vi "Projeto.vi"(8 "Error In":errorcluster) -> (0 "Error Out":errorcluster)   [LabVIEW 2014]
uses:
  Aquisicao de Dados.lvlib
  <vilib>/express/express analysis/Spectral/XNode/ExpressSpectralMeasurementsBlockNode.xnode
  <vilib>/express/express analysis/Spectral/Block/exnSpectralBlock spectral measurements RMS poly.vi
  <vilib>/express/express analysis/Spectral/Block/exnSpectralBlock spectral measurements RMS WFM.vi
  <vilib>/measure/NI_MAPro.lvlib
  <vilib>/measure/matone.llb/Extract Multiple Tone Information 1 Chan.vi
panel:
  out "resolução espectral":dbl
  out "V/2^n":dbl
  out "Período de amostragem":dbl
  out "multiple tone information":T1(array[cluster]) {"detected phase (deg)" format="%_6g"; "detected amplitude" format="%_6p"; "detected frequency" format="%_6p"}
  out "frequência de amostragem":dbl
  out "período de amostragem":dbl
  out "amostras janelada":i32
  out "amostras total":i32
  out "Waveform Graph 3":cluster{"f0":dbl, "df":dbl, "magnitude":dbl[]}(graph)
  out "mín local":dbl
  out "máx local":dbl
  out "min global":dbl
  out "max global":dbl
  out "Waveform Graph 2":cluster{"f0":dbl, "df":dbl, "magnitude":dbl[]}(graph)
  out "Waveform Graph":waveform(dbl)(graph)
  in  "stop":bool
  out "Canal 1":waveform(dbl)(graph)
  out "Canal 0":waveform(dbl)(graph)
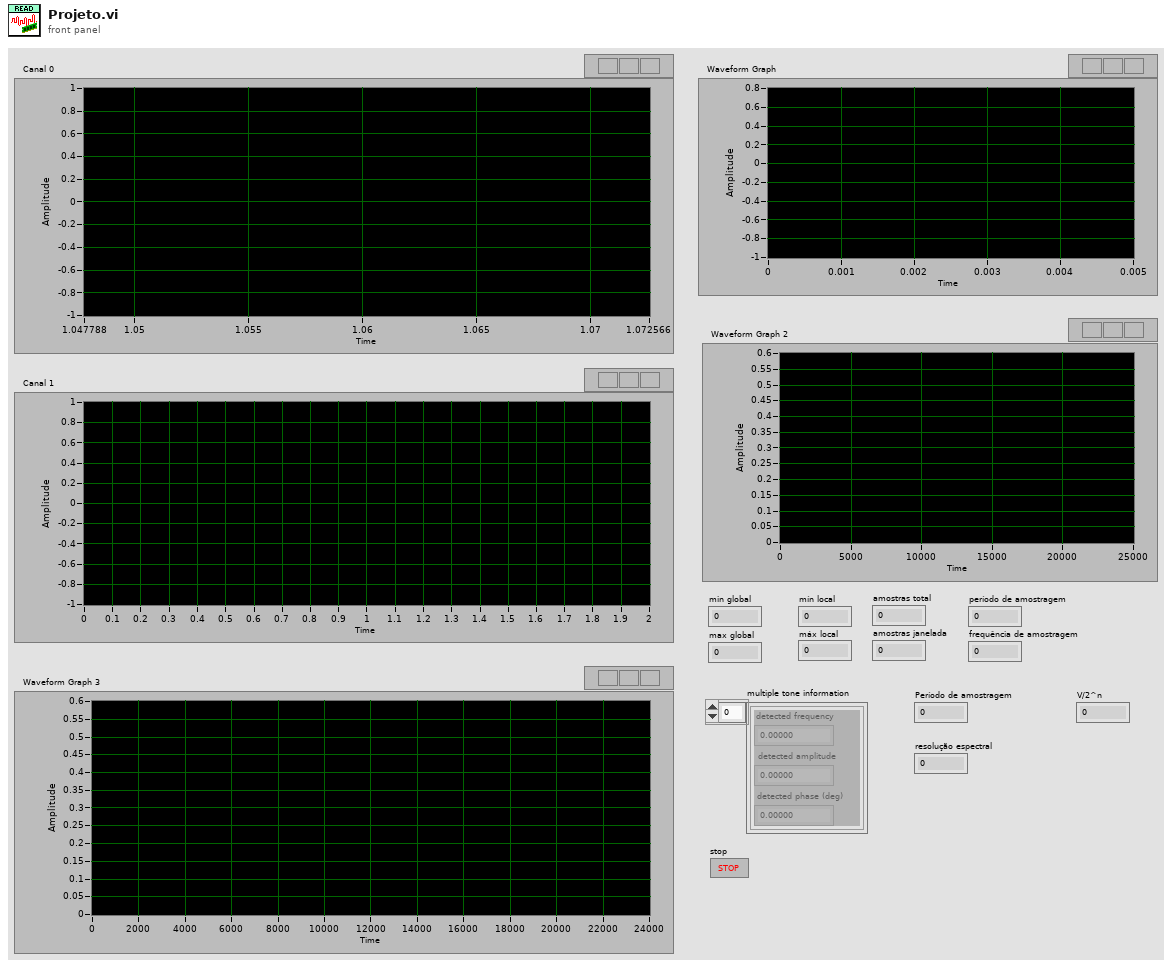
[diagram p1: front panel]
types:
  T1 = cluster{"detected frequency":dbl, "detected amplitude":dbl, "detected phase (deg)":dbl}[]
  T2 = enum32{".WAV File", "LTSpice Simulation", "Microphone", "MultiSim Simulation", "Serial Port"}
  T3 = typedef "Aquisicao de Dados.lvlib/_ACC_DATA_ Config DAta State.ctl" = cluster{"_RAW_ Traces":cluster{"Trace Name":string, "Trace Type":string, "Trace Raw Data":dbl[], "Trace Waveform":waveform(dbl)}[], "_WAV_ Traces":waveform(dbl)[], "_MIC_ Config":cluster{"task ID":T4, "Data Chunk Size":i32, "Num Channels":i32, "Resolution":i32, "Sampling Frequency":dbl, "device ID":u32, "Num Chunks":i32}, "_LVM_ Traces":cluster{"Trace Name":string, "Trace Type":string, "Trace Raw Data":dbl[], "Trace Waveform":waveform(dbl)}[]}
  T4 = typedef "Sound Input Task ID.ctl" = u32
  T5 = cluster{"averaging mode":u16, "weighting mode":u16, "number of averages":u32}
  T6 = cluster{"dB On (F)":bool, "unwrap phase (F)":bool, "convert to degree (F)":bool}
  T7 = typedef "LVCursorListTypeDef.ctl" = cluster{"Name":string, "Color":u32, "Style":u8, "Point Style":u8, "Name Visible":bool, "Allow Drag":bool, "Cursor Mode":u32, "Plot":i32, "Index":i32, "Position":cluster{"X":dbl, "Y":dbl}, "X Scale":u32, "Y Scale":u32, "Watch Plots":i32[], "Watch All Plots":bool, "Plot Area":i32, "Label Offset":cluster{"X":dbl, "Y":dbl}}[]
  T8 = cluster{"Name":string, "Color":u32, "Style":u8, "Point Style":u8, "Name Visible":bool, "Allow Drag":bool, "Cursor Mode":u32, "Plot":i32, "Index":i32, "Position":cluster{"X":dbl, "Y":dbl}, "X Scale":u32, "Y Scale":u32, "Watch Plots":i32[], "Watch All Plots":bool, "Plot Area":i32, "Label Offset":cluster{"X":dbl, "Y":dbl}}
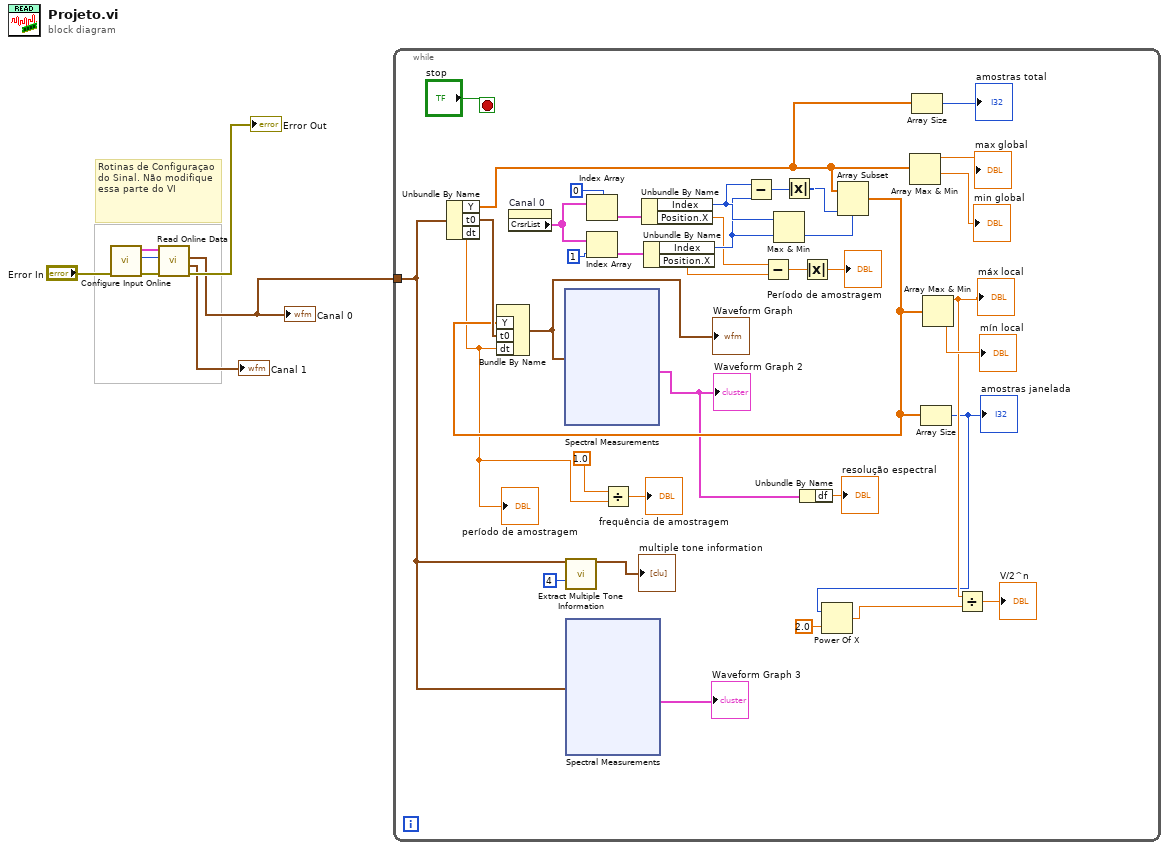
[diagram p0: block diagram]
diagram:
  # "Rotinas de Configuraçao do Sinal. Não modifique essa parte do VI"
  n1 = call "Configure Input Online.vi"("Error In"="Error In") -> ("Error Out"=w7:errorcluster, "Metodo de Entrada"=w5:T2, "Config Out"=w3:T3)  [unwired: 8 in]
  n2 = call "Read Online Data.vi"("Error In"=w7, "Metodo de Entrada"=w5, "Config Out"=w3) -> ("Error Out"=→"Error Out":errorcluster, "Channel 1"=→"Canal 1":waveform(dbl), "Channel 0"=w1:waveform(dbl))  [unwired: 6 in]
  "Canal 0" <- w1
  n3 = while {
    tunnel: w1 -> [w24]
    stop <- "stop" stop-if-true
    n4 = Unbundle By Name(w24) -> ("Y"=w29:dbl[], "t0"=w43:timestamp, "dt"=w26:dbl)
    "período de amostragem" <- w26
    n5 = property on="Canal 0" class="WFGraph (strict)"() -> ("CrsrList"=w40:T7)  [unwired: 2 in, 2 out]
    n6 = call-poly <vilib>:"Extract Multiple Tone Information.vi"("time signal in"=w24, "max num tones"=4) -> ("multiple tone information"=→"multiple tone information":T1)  [unwired: 11 in, 2 out]
    n7 = xnode "Spectral Measurements"("Signals"=w24) -> ("FFT - (RMS)"=→"Waveform Graph 3":cluster{"f0":dbl, "df":dbl, "magnitude":dbl[]})  [unwired: 1 in, 2 out]
    n8 = Index Array(array=w40, index=0) -> (element=w34:T8)
    n9 = Index Array(array=w40, index=1) -> (element=w21:T8)
    n10 = Divide(x=1.0, y=w26) -> (x/y=→"frequência de amostragem":dbl)
    n11 = Unbundle By Name(w34) -> ("Index"=w38:i32, "Position.X"=w20:dbl)
    n12 = Unbundle By Name(w21) -> ("Index"=w37:i32, "Position.X"=w19:dbl)
    n13 = Subtract(x=w38, y=w37) -> (x-y=w36:i32)
    n14 = Subtract(x=w20, y=w19) -> (x-y=w18:dbl)
    n15 = Max & Min(x=w38, y=w37) -> (min(x,y)=w39:i32)  [unwired: 1 out]
    n16 = Absolute Value(x=w36) -> (abs(x)=w35:i32)
    n17 = Absolute Value(x=w18) -> (abs(x)=→"Período de amostragem":dbl)
    n18 = Array Subset(array=w29, index=w39, length=w35) -> (w28:dbl[])
    n19 = Bundle By Name("Y"=w28, "t0"=w43, "dt"=w26) -> (w33:waveform(dbl))  [unwired: 1 in]
    "Waveform Graph" <- w33
    n20 = xnode "Spectral Measurements"("Signals"=w33) -> ("FFT - (RMS)"=w9:cluster{"f0":dbl, "df":dbl, "magnitude":dbl[]})  [unwired: 1 in, 2 out]
    "Waveform Graph 2" <- w9
    n21 = Unbundle By Name(w9) -> ("df"=→"resolução espectral":dbl)
    n22 = Array Max & Min(array=w29) -> (max value=→"max global":dbl, min value=→"min global":dbl)  [unwired: 2 out]
    n23 = Array Size(array=w29) -> (size(s)=→"amostras total":i32)
    n24 = Array Size(array=w28) -> (size(s)=w10:i32)
    "amostras janelada" <- w10
    n25 = Power Of X(1:2.0 ("x"), 2:w10) -> (0:w15:dbl)
    n26 = Array Max & Min(array=w28) -> (max value=w12:dbl, min value=→"mín local":dbl)  [unwired: 2 out]
    "máx local" <- w12
    n27 = Divide(x=w12, y=w15) -> (x/y=→"V/2^n":dbl)
  }
